vi "Intrinsic Imager.vi"() -> ()   [LabVIEW 2014]
uses:
  <vilib>/vision/Image Controls.llb/IMAQ Image.ctl
  <instrlib>/niHWS/nihws.llb/niHWS Open File Permissions ID.ctl
  <vilib>/Utility/error.llb/DialogType.ctl
  <vilib>/DAQmx/read.llb/DAQmx Read (Analog Wfm 1Chan NSamp).vi
  <vilib>/Analysis/baseanly.llb/Mean (DBL).vi
  <instrlib>/niHWS/nihws.llb/niHWS Write Analog DBL.vi
  <vilib>/DAQmx/miscellaneous.llb/DAQmx Fill In Error Info.vi
  <instrlib>/niHWS/nihws.llb/niHWS Write Analog WDT.vi
  <instrlib>/niHWS/nihws.llb/niHWS Write Digital 2D U16.vi
  <vilib>/vision/NI_Vision_Development_Module.lvlib
  <resource>/objmgr/daqmx.rc
  <vilib>/Analysis/NI_AALBase.lvlib
panel:
  in  "Single trial":bool
  in  "Analysis":enum32{"Amp", "Angle", "Amp/Angle"}(radio)
  in  "Analyze":bool
  in  "Period (ms)":dbl=16641.0
  in  "Pixel Thr":dbl=4095.0
  in  "Magnify":bool
  in  "PseudoColor":bool
  out "Frames":u32 caption="Image Number"
  out "Rep. Fps":dbl caption="Frame Rate"
  out "Fps":dbl
  out "Ephys Rate":dbl=1000.0
  in  "Final res.":dbl=512.0
  out "Image Parameters : Bits per Pixel":u32
  out "Numeric":i32
  out "Setup":i32
  out "PPhocus?":bool
  out "file handle out":u32
  out "Recording":bool
  in  "stop":bool
  out "Raw Image":T1(plugin-control)
  out "Rec Time":dbl
  out "Photodiode display":waveform(dbl)(graph)
  in  "Recording Path":path
  in  "Rec":bool
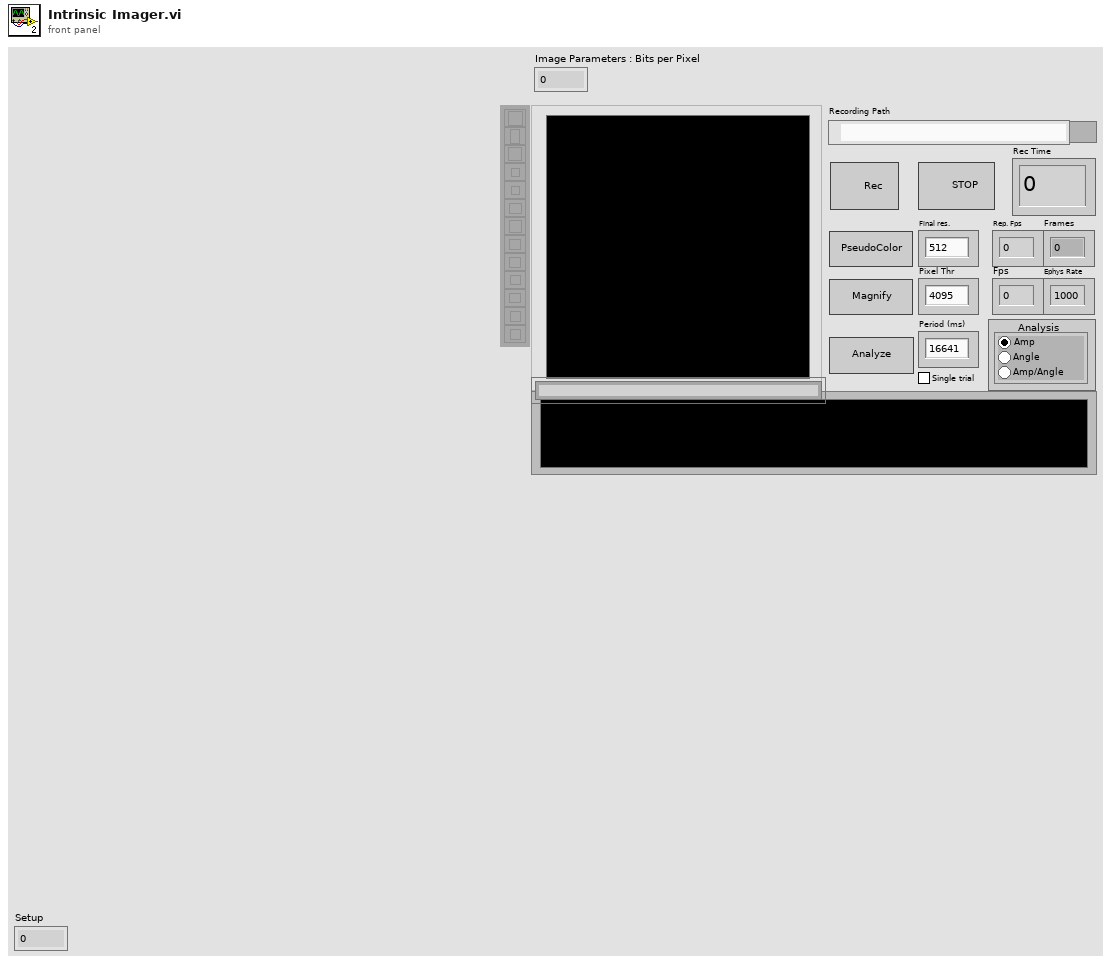
[diagram p1: front panel]
types:
  T1 = typedef "IMAQ Image.ctl" = refnum<image>
  T2 = typedef "niHWS Open File Permissions ID.ctl" = enum32{"Read Only", "Read/Write Existing", "Read/Write/Create New", "Read/Write/Create New Always"}
  T3 = enum32{"Average", "Min", "Max", "Clear  if < ", "Clear  if < or =", "Clear  if =", "Clear  if > or =", "Clear  if >"}
  T4 = enum32{"Invalid", "Standard", "Closed", "Hidden", "Minimized", "Maximized"}
  T5 = typedef "Image Type" = u32
  T6 = cluster{"IMAQ Session Out":refnum<k11>, "New Image":T1, "error out":errorcluster, cluster{dbl, i32}[], "New Image":T1}
  T7 = cluster{"IMAQ Session Out":refnum<k11>, "Image Out":T1, "error out":errorcluster, cluster{dbl, i32}[], "New Image":T1}
  T8 = typedef "DialogType.ctl" = u16
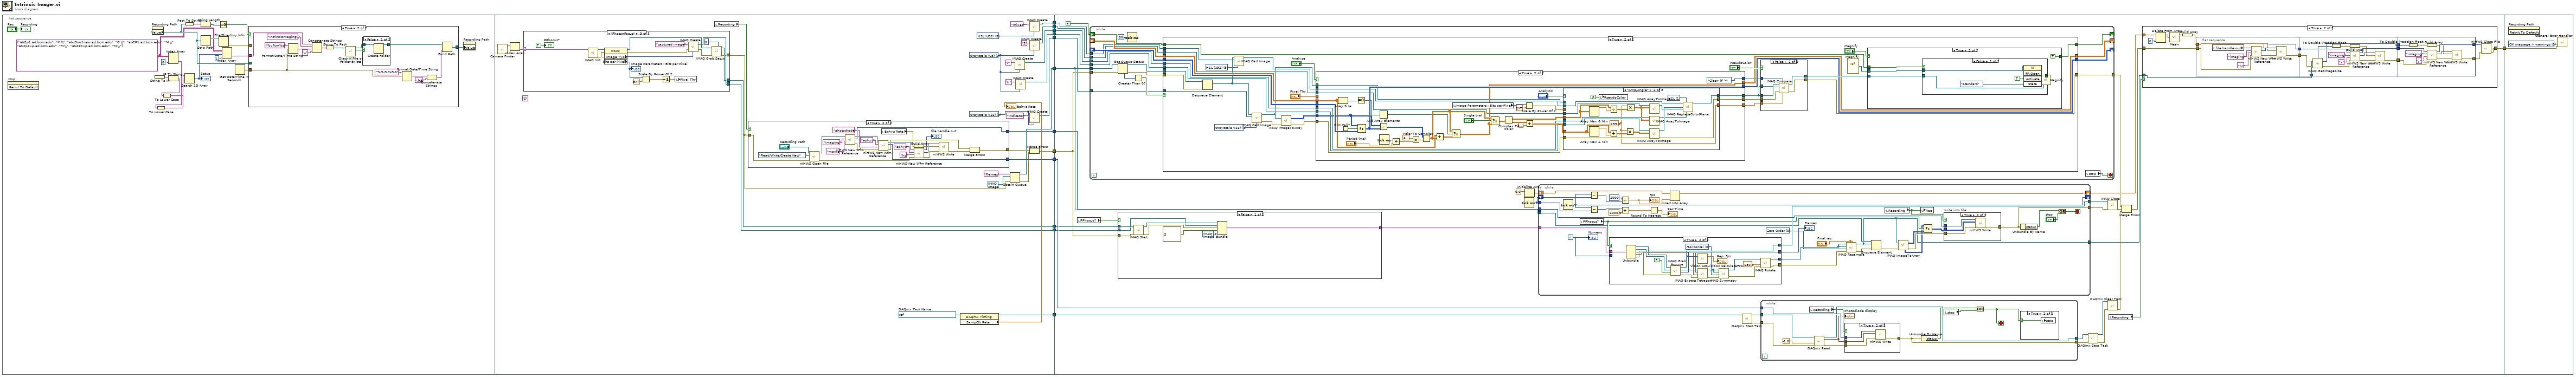
[diagram p0: block diagram]
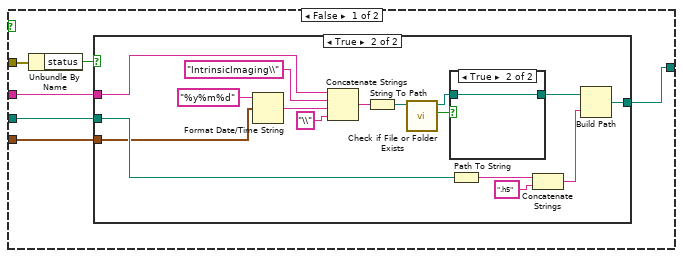
[diagram p2: hidden frame]
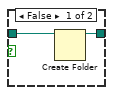
[diagram p4: hidden frame]
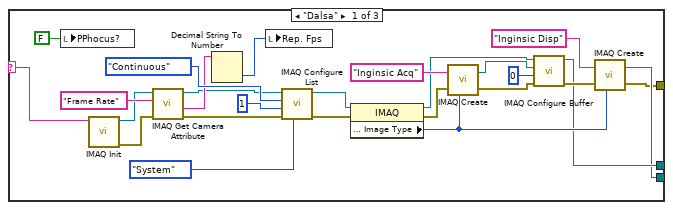
[diagram p6: hidden frame]
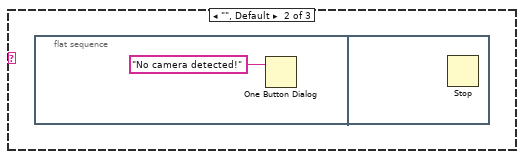
[diagram p7: hidden frame]
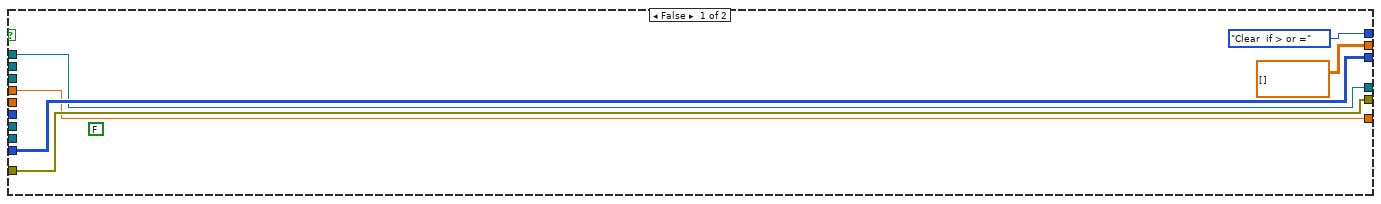
[diagram p10: hidden frame]
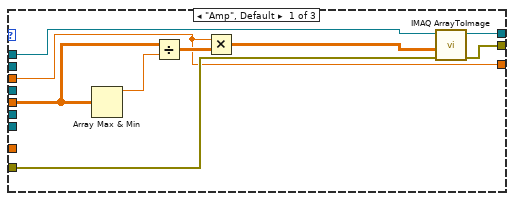
[diagram p11: hidden frame]
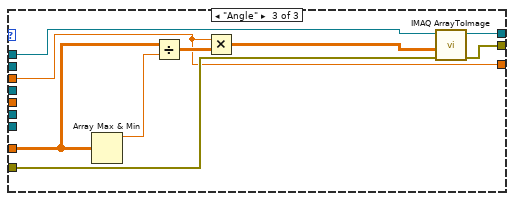
[diagram p12: hidden frame]
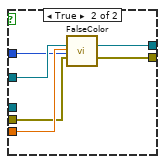
[diagram p13: hidden frame]
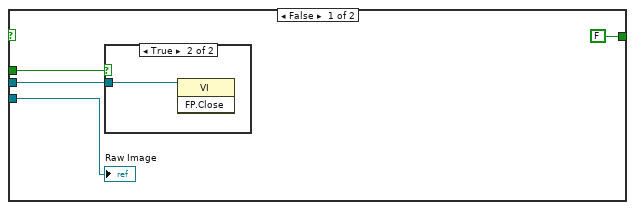
[diagram p14: hidden frame]
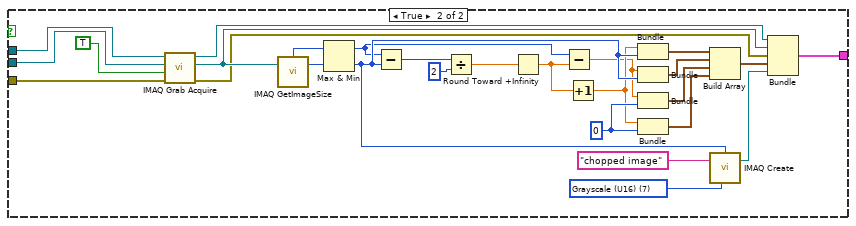
[diagram p17: hidden frame]
diagram:
  n1 = flat-sequence {
    tunnel: [w107] -> w13
    tunnel: [w106] -> w12
    tunnel: [w100] -> w10
    tunnel: [w104] -> w9
    tunnel: [w101] -> w8
    tunnel: [w92] -> w7
    tunnel: [w91] -> w6
    tunnel: [w88] -> w5
    tunnel: [w86] -> w4
    tunnel: [w84] -> w3
    tunnel: [w83] -> w2
    tunnel: [w79] -> w1
    tunnel: w13 -> [w203]
    tunnel: w12 -> [w204]
    tunnel: [w202] -> w11
    tunnel: w10 -> [w193]
    tunnel: w9 -> [w194]
    tunnel: w8 -> [w185]
    tunnel: w7 -> [w182]
    tunnel: w6 -> [w183]
    tunnel: w5 -> [w180]
    tunnel: w4 -> [w179]
    tunnel: w3 -> [w178]
    tunnel: w2 -> [w177]
    tunnel: w1 -> [w176]
    tunnel: w11 -> [w551]
    frame #0 {
      w19 = string[][] [["at-2p1.ad.bcm.edu", "M:\\"], ["at-s5no1new.ad.bcm.edu", "G:\\"], ["at-2P1.ad.bcm.edu", "M:\\"], ["at-2p1xp.ad.bcm.edu", "M:\\"], ["at-2P1xp.ad.bcm.edu", "M:\\"]]
      n2 = invoke on="stop" class="Bool (strict)" method="Reinit To Default"() -> ()  [unwired: 3 in, 3 out]
      n3 = property on="Recording Path" class="Path"() -> ("Value"=w26:path)  [unwired: 2 in, 2 out]
      n4 = String To IP() -> (0:w23:u32)  [unwired: 1 in]
      n5 = IP To String(2:w23) -> (0:w15:string)  [unwired: 1 in]
      n6 = To Lower Case(string=w15) -> (all lower case string=w14:string)
      n7 = Index Array(array=w19, index (col)=0 ("disabled index (col)")) -> (element=w17:string[])  [unwired: 1 in]
      n8 = To Lower Case(string=w17) -> (all lower case string=w16:string[])
      n9 = Path To String(path=w26) -> (string=w31:string)
      n10 = Search 1D Array(1D array=w16, element=w14) -> (index of element=w20:i32)  [unwired: 1 in]
      "Setup" <- w20
      n11 = String Length(string=w31) -> (length=w30:i32)
      n12 = Strip Path(path=w26) -> (stripped path=w25:path)  [unwired: 1 out]
      n13 = Equal To 0?(x=w30) -> (x = 0?=w29:bool)
      n14 = File/Directory Info(path=w25) -> (error out=w24:errorcluster)  [unwired: 1 in, 6 out]
      n15 = Index Array(array=w19, index (row)=w20, index (col)=1 ("disabled index (col)")) -> (element=w18:string)
      n16 = Get Date/Time In Seconds() -> (seconds since 1Jan1904=w32:timestamp)
      n17 = case shown="True" w29 {
        tunnel: w32 -> [w36 w65]
        tunnel: w26 -> [w37 _]
        tunnel: [w38 w63] -> w28
        tunnel: w24 -> [w34 _]
        tunnel: w18 -> [w33 w59]
        frame False {
          n18 = Unbundle By Name(w34) -> ("status"=w35:bool)
          n19 = case shown="True" w35 {
            tunnel: [w39 w46] -> w38
            tunnel: w37 -> [w39 w45]
            tunnel: w36 -> [_ w41]
            tunnel: w33 -> [_ w40]
            frame False {
            }
            frame True {
              n20 = Format Date/Time String(time format string (%c)="%y%m%d", seconds (now)=w41) -> (date/time string=w50:string)  [unwired: 1 in]
              n21 = Concatenate Strings(w40, "IntrinsicImaging\\", w50, "\\") -> (w49:string)
              n22 = String To Path(string=w49) -> (path=w55:path)
              n23 = call <vilib>:"Check if File or Folder Exists.vi"("path"=w55) -> ("file or folder exists?"=w53:bool, "dup path"=w52:path)  [unwired: 8 in, 1 out]
              n24 = case shown="True" w53 {
                tunnel: [w57 w58] -> w54
                tunnel: w52 -> [w56 w58]
                frame False {
                  n25 = Create Folder(path (use dialog)=w56) -> (created path=w57:path)  [unwired: 2 in, 2 out]
                }
                frame True {
                }
              }
              n26 = Path To String(path=w45) -> (string=w42:string)
              n27 = Concatenate Strings(w42, ".h5" ("string")) -> (w43:string)
              n28 = Build Path(base path=w54, name or relative path=w43) -> (appended path=w46:path)
            }
          }
        }
        frame True {
          n29 = Format Date/Time String(time format string (%c)="%y%m%d", seconds (now)=w65) -> (date/time string=w71:string)  [unwired: 1 in]
          n30 = Concatenate Strings(w59, "IntrinsicImaging\\", w71, "\\") -> (w72:string)
          n31 = String To Path(string=w72) -> (path=w64:path)
          n32 = call <vilib>:"Check if File or Folder Exists.vi"("path"=w64) -> ("file or folder exists?"=w68:bool, "dup path"=w69:path)  [unwired: 8 in, 1 out]
          n33 = case shown="False" w68 {
            tunnel: [w76 w77] -> w67
            tunnel: w69 -> [w75 w77]
            frame False {
              n34 = Create Folder(path (use dialog)=w75) -> (created path=w76:path)  [unwired: 2 in, 2 out]
            }
            frame True {
            }
          }
          n35 = Format Date/Time String(time format string (%c)="%H-%M-%S", seconds (now)=w65) -> (date/time string=w62:string)  [unwired: 1 in]
          n36 = Concatenate Strings(w62, ".h5" ("string")) -> (w60:string)
          n37 = Build Path(base path=w67, name or relative path=w60) -> (appended path=w63:path)
        }
      }
      n38 = property on="Recording Path" class="Path"("Value"=w28) -> ()  [unwired: 2 in, 2 out]
      "Recording" <- "Rec"
    }
    frame #1 {
      w80 = T5 1 items=["Grayscale (U8)", "Grayscale (I16)", "Grayscale (SGL)", "Complex (CSG)", "RGB (U32)", "HSL (U32)", "RGB (U64)", "Grayscale (U16)"] ("Image Type")
      (unwired) "S" ("Image Name")
      w82 = T5 0 items=["Grayscale (U8)", "Grayscale (I16)", "Grayscale (SGL)", "Complex (CSG)", "RGB (U32)", "HSL (U32)", "RGB (U64)", "Grayscale (U16)"] ("Image Type")
      w89 = T5 5 items=["Grayscale (U8)", "Grayscale (I16)", "Grayscale (SGL)", "Complex (CSG)", "RGB (U32)", "HSL (U32)", "RGB (U64)", "Grayscale (U16)"] ("Image Type")
      w103 = refnum<k21> "Photodiode Intrinsic Imaging"  # DAQmx Task Name
      n39 = call "Camera Finder.vi"() -> ("IMAQ Interfaces"=w98:string[])  [unwired: 11 in]
      n40 = Index Array(array=w98) -> (element=w99:string)  [unwired: 1 in]
      n41 = case shown="\"PhotonFocus\"" w99 {
        selector: w99 -> [w111 _ w140]
        tunnel: [w114 _ w143] -> w104
        tunnel: [w115 _ w142] -> w100
        tunnel: [w113 _ w141] -> w95
        frame "Dalsa" {
          n42 = local write "PPhocus?"(FALSE ("PPhocus?")) -> ()
          n43 = call <vilib>:"IMAQ Init.vi"("Interface Name"=w111) -> ("error out"=w116:errorcluster, "IMAQ Session Out"=w117:refnum<k11>)  [unwired: 9 in]
          n44 = call <vilib>:"IMAQ Get Camera Attribute.vi"("error in (no error)"=w116, "Camera Attribute"="Frame Rate", "IMAQ Session In"=w117) -> ("error out"=w108:errorcluster, "Attribute Value"=w110:string, "IMAQ Session Out"=w109:refnum<k11>)  [unwired: 4 in]
          n45 = Decimal String To Number(string=w110) -> (number=w112:i32)  [unwired: 2 in, 1 out]
          n46 = local write "Rep. Fps"(w112) -> ()
          n47 = call <vilib>:"IMAQ Configure List.vi"("Memory Location"=enum16{"System", "Onboard"}."System", "error in (no error)"=w108, "Number of buffers"=u32 1, "Continuous?"=enum16{"One-Shot", "Continuous"}."Continuous" ("Continuous ?"), "IMAQ Session In"=w109) -> ("error out"=w125:errorcluster, "IMAQ Session Out"=w126:refnum<k11>)  [unwired: 5 in]
          n48 = property class="IMAQ"(reference=w126, error in=w125) -> (reference out=w124:refnum<k11>, error out=w123:errorcluster, "Image Parameters : Image Type"=w122:u32)
          n49 = call "IMAQ Create"("Image Name"="Inginsic Acq", "Image Type"=w122, "error in (no error)"=w123) -> ("New Image"=w119:T1, "error out"=w129:errorcluster)  [unwired: 2 in]
          n50 = call <vilib>:"IMAQ Configure Buffer.vi"("error in (no error)"=w129, "Buffer Number"=u32 0, "Image In"=w119, "IMAQ Session In"=w124) -> ("error out"=w121:errorcluster, "IMAQ Session Out"=w115:refnum<k11>)  [unwired: 6 in]
          n51 = call "IMAQ Create"("Image Name"="Inginsic Disp", "Image Type"=w122, "error in (no error)"=w121) -> ("New Image"=w114:T1, "error out"=w113:errorcluster)  [unwired: 2 in]
        }
        frame "", Default {
          n52 = flat-sequence {
            frame #0 {
              n53 = One Button Dialog(message="No camera detected!" ("error source (\" \")")) -> ()  [unwired: 1 in, 1 out]
            }
            frame #1 {
              n54 = Stop() -> ()  [unwired: 1 in]
            }
          }
        }
        frame "PhotonFocus" {
          n55 = call <vilib>:"IMAQ Init.vi"("Interface Name"=w140) -> ("error out"=w150:errorcluster, "IMAQ Session Out"=w149:refnum<k11>)  [unwired: 1 in, 8 out]
          n56 = property class="IMAQ"(reference=w149, error in=w150) -> (reference out=w144:refnum<k11>, error out=w147:errorcluster, "Image Parameters : Image Type"=w148:u32, "Bits per Pixel"=w138:u32)
          "Image Parameters : Bits per Pixel" <- w138
          n57 = Scale By Power Of 2(n=w138, x=ext 1.0) -> (x*2^n=w136:ext)
          n58 = Decrement(x=w136) -> (x-1=w135:ext)
          n59 = local write "Pixel Thr"(w135) -> ()
          n60 = call "IMAQ Create"("Image Name"="captured image", "Image Type"=w148, "error in (no error)"=w147) -> ("New Image"=w143:T1, "error out"=w145:errorcluster)  [unwired: 1 in, 1 out]
          n61 = call <vilib>:"IMAQ Grab Setup.vi"("Channel"=0, "error in (no error)"=w145, "IMAQ Session In"=w144) -> ("error out"=w141:errorcluster, "IMAQ Session Out"=w142:refnum<k11>)  [unwired: 7 out]
          "PPhocus?" <- TRUE ("PPhocus?")
        }
      }
      n62 = local read "Recording"() -> (w105:bool)
      n63 = case shown="True" w105 {
        tunnel: [_ w175] -> w107
        tunnel: [_ w155] -> w94
        tunnel: [_ w173] -> w106
        tunnel: w95 -> [_ w152]
        frame False {
        }
        frame True {
          n64 = call <instrlib>:"niHWS Open File.vi"("error in (no error)"=w152, "permissions (0:read only)"=niHWS_Open_File_Permissions_ID."Read/Write/Create New", "file path"="Recording Path") -> ("error out"=w170:errorcluster, "file handle"=w162:u32)  [unwired: 7 in]
          n65 = call <instrlib>:"niHWS New Wfm Reference.vi"("waveform name (empty)"="movie" ("format string"), "group name (empty)"="imaging", "file handle in"=w162) -> ("error out"=w158:errorcluster, "waveform reference"=w175:u32, "file handle out"=w159:u32)  [unwired: 6 in]
          n66 = call <instrlib>:"niHWS New Wfm Reference.vi"("error in (no error)"=w158, "waveform name (empty)"="photodiode", "group name (empty)"="ephys", "file handle in"=w159) -> ("error out"=w157:errorcluster, "waveform reference"=w173:u32, "file handle out"=w174:u32)  [unwired: 5 in]
          n67 = local read "Ephys Rate"() -> (w153:dbl)
          n68 = Build Array(w153) -> (w166:dbl[])
          n69 = call <instrlib>:"niHWS New Wfm Reference.vi"("error in (no error)"=w170, "waveform name (empty)"="hz" ("group name (empty)"), "group name (empty)"="ephys", "file handle in"=w174) -> ("error out"=w165:errorcluster, "waveform reference"=w169:u32, "file handle out"=→"file handle out":u32)  [unwired: 5 in]
          n70 = call-poly <instrlib>:"niHWS Write.vi"("error in (no error)"=w165, "data"=w166, "waveform reference in"=w169) -> ("error out"=w156:errorcluster)  [unwired: 7 in, 1 out]
          n71 = Merge Errors(w157, w156) -> (w155:errorcluster)
        }
      }
      n72 = property class="DAQmx Timing"(reference=w103) -> (reference out=w101:refnum<k21>, "SampClk.Rate"=→"Ephys Rate":dbl)  [unwired: 1 in, 1 out]
      n73 = Obtain Queue(name (unnamed)="Frames", element data type=T1 refnum ("New Image"), error in (no error)=w95) -> (queue out=w91:refnum<queue>, error out=w93:errorcluster)  [unwired: 2 in, 1 out]
      n74 = call "IMAQ Create"("Image Name"="V", "Image Type"=w82) -> ("New Image"=w86:T1)  [unwired: 3 in, 1 out]
      n75 = call "IMAQ Create"("Image Name"="H", "Image Type"=w82) -> ("New Image"=w84:T1)  [unwired: 3 in, 1 out]
      n76 = call "IMAQ Create"("Image Name"="mixed", "Image Type"=w89) -> ("New Image"=w88:T1)  [unwired: 3 in, 1 out]
      n77 = call "IMAQ Create"("Image Name"="S", "Image Type"=w82) -> ("New Image"=w83:T1)  [unwired: 3 in, 1 out]
      n78 = call "IMAQ Create"("Image Name"="Indicator", "Image Type"=w80) -> ("New Image"=w79:T1)  [unwired: 3 in, 1 out]
      n79 = Merge Errors(w94, w93) -> (w92:errorcluster)
    }
    frame #2 {
      n80 = local read "PPhocus?"() -> (w187:bool)
      n81 = while {
        shift-right: [w228] -> _
        shift-left: FALSE -> [w227]
        tunnel: w183 -> [w225]
        tunnel: w182 -> [w221]
        tunnel: [w219] -> w181
        shift-right: [w218] -> _
        shift-left: _ -> [w217]
        shift-right: [w216] -> _
        shift-left: _ -> [w215]
        tunnel: w180 -> [w214]
        tunnel: w179 -> [w213]
        tunnel: w178 -> [w212]
        tunnel: w177 -> [w211]
        tunnel: w176 -> [w210]
        stop <- w229 stop-if-true
        n82 = Get Queue Status(queue=w225, error in (no error)=w221) -> (queue out=w222:refnum<queue>, error out=w220:errorcluster, # elements in queue=w224:i32)  [unwired: 1 in, 5 out]
        n83 = Wait (ms)(milliseconds to wait=u32 50) -> ()  [unwired: 1 out]
        n84 = Greater Than 0?(x=w224) -> (x > 0?=w223:bool)
        n85 = case shown="True" w223 {
          tunnel: [w233 w263] -> w228
          tunnel: w227 -> [w233 w262]
          tunnel: w222 -> [_ w259]
          tunnel: w220 -> [w232 w258]
          tunnel: [w232 w256] -> w219
          tunnel: [w231 w254] -> w218
          tunnel: w217 -> [w231 w253]
          tunnel: [w230 w252] -> w216
          tunnel: w215 -> [w230 w251]
          tunnel: w214 -> [_ w238]
          tunnel: w213 -> [_ w237]
          tunnel: w212 -> [_ w236]
          tunnel: w211 -> [_ w235]
          tunnel: w210 -> [_ w234]
          frame False {
          }
          frame True {
            w240 = T5 5 items=["Grayscale (U8)", "Grayscale (I16)", "Grayscale (SGL)", "Complex (CSG)", "RGB (U32)", "HSL (U32)", "RGB (U64)", "Grayscale (U16)"] ("Image Type")
            w242 = T5 1 items=["Grayscale (U8)", "Grayscale (I16)", "Grayscale (SGL)", "Complex (CSG)", "RGB (U32)", "HSL (U32)", "RGB (U64)", "Grayscale (U16)"] ("Image Type")
            n86 = Dequeue Element(queue=w259, error in (no error)=w258) -> (element=w241:T1)  [unwired: 1 in, 3 out]
            n87 = call "IMAQ Cast Image"("Image Type"=w240, "Image Dst"=w238, "Image Src"=w241) -> ("Image Dst Out"=w239:T1)  [unwired: 7 in, 1 out]
            n88 = call "IMAQ Cast Image"("Image Type"=w242, "Image Dst"=w234, "Image Src"=w241) -> ("error out"=w248:errorcluster, "Image Dst Out"=w250:T1)  [unwired: 7 in]
            n89 = call "IMAQ ImageToArray"("error in (no error)"=w248, "Image"=w250) -> ("error out"=w247:errorcluster, "Image Pixels (I16)"=w255:i16[][])  [unwired: 2 in, 3 out]
            n90 = case shown="True" "Analyze" {
              tunnel: w255 -> [w271 w306]
              tunnel: [w271 w305] -> w254
              tunnel: w253 -> [_ w307]
              tunnel: [cdb[][] [] w276] -> w252
              tunnel: w251 -> [_ w280]
              tunnel: w250 -> [w270 w295]
              tunnel: [w270 w294] -> w249
              tunnel: w247 -> [w269 w292]
              tunnel: [w269 w293] -> w246
              tunnel: [w268 w286] -> w245
              tunnel: "Pixel Thr" -> [w268 _]
              tunnel: [T3."Clear  if > or =" ("Operator") T3."Clear  if >" ("Operator")] -> w243
              tunnel: w239 -> [_ w275]
              tunnel: w236 -> [_ w274]
              tunnel: w235 -> [_ w273]
              tunnel: w237 -> [_ w272]
              frame False {
                (unwired) FALSE
              }
              frame True {
                n91 = Array Size(array=w280) -> (size(s)=w279:i32[])
                n92 = First Call?() -> (First Call?: T/F=w308:bool)
                n93 = Equal To 0?(x=w279) -> (x = 0?=w278:bool[])
                n94 = Select(t=w306, s=w308, f=w307) -> (s? t:f=w305:i16[][])
                n95 = And Array Elements(Boolean array=w278) -> (logical AND=w277:bool)
                n96 = Subtract(x=w306, y=w305) -> (x-y=w299:i16[][])
                n97 = Tick Count (ms)() -> (millisecond timer value=w302:u32)
                n98 = Divide(x=w302, y="Period (ms)") -> (x/y=w300:dbl)
                n99 = Multiply(x=6.283185307179586, y=w300) -> (x*y=w304:dbl)
                n100 = Polar To Complex(1:w304, 2:w299) -> (0:w281:cdb[][])
                n101 = Add(x=w280, y=w281) -> (x+y=w282:cdb[][])
                n102 = Select(t=w281, s=w277, f=w282) -> (s? t:f=w276:cdb[][])
                n103 = local read "Image Parameters : Bits per Pixel"() -> (w288:u32)
                n104 = Select(t=w281, s="Single trial", f=w276) -> (s? t:f=w283:cdb[][])
                n105 = Complex To Polar(r * e^(i*theta)=w283) -> (r=w291:dbl[][], theta=w298:dbl[][])
                n106 = Scale By Power Of 2(n=w288, x=ext 1.0) -> (x*2^n=w287:ext)
                n107 = Add(x=w298, y=3.141592653589793) -> (x+y=w290:dbl[][])
                n108 = case shown="\"Amp/Angle\"" "Analysis" {
                  tunnel: w295 -> [w309 _ w344]
                  tunnel: [w315 w330 w341] -> w294
                  tunnel: [w314 w333 w342] -> w293
                  tunnel: w292 -> [w313 w334 w343]
                  tunnel: w291 -> [w312 w318 _]
                  tunnel: w290 -> [_ w319 w345]
                  tunnel: w287 -> [w311 _ w340]
                  tunnel: [w311 w320 w340] -> w286
                  tunnel: w275 -> [_ w331 _]
                  tunnel: w274 -> [_ w326 _]
                  tunnel: w273 -> [_ w325 _]
                  tunnel: w272 -> [_ w323 _]
                  frame "Amp", Default {
                    n109 = Array Max & Min(array=w312) -> (max value=w316:dbl)  [unwired: 3 out]
                    n110 = Divide(x=w312, y=w316) -> (x/y=w317:dbl[][])
                    n111 = Multiply(x=w311, y=w317) -> (x*y=w310:ext[][])
                    n112 = call "IMAQ ArrayToImage"("error in (no error)"=w313, "Image Pixels (I16)"=w310, "Image"=w309) -> ("error out"=w314:errorcluster, "Image Out"=w315:T1)  [unwired: 7 in]
                  }
                  frame "Amp/Angle" {
                    w332 = u16 1 items=["RGB", "HSL", "HSV", "HSI"] ("Color Mode")
                    w320 = 255.0
                    n113 = Array Max & Min(array=w318) -> (max value=w336:dbl)  [unwired: 3 out]
                    n114 = Array Max & Min(array=w319) -> (max value=w337:dbl)  [unwired: 3 out]
                    n115 = local write "PseudoColor"(FALSE ("PseudoColor")) -> ()
                    n116 = Divide(x=w318, y=w336) -> (x/y=w335:dbl[][])
                    n117 = Divide(x=w319, y=w337) -> (x/y=w338:dbl[][])
                    n118 = Multiply(x=w320, y=w338) -> (x*y=w328:dbl[][])
                    n119 = Multiply(x=w320, y=w335) -> (x*y=w322:dbl[][])
                    n120 = call "IMAQ ArrayToImage"("Image Pixels (U8)"=w322, "Image"=w325) -> ("Image Out"=w324:T1)  [unwired: 8 in, 1 out]
                    n121 = call "IMAQ ArrayToImage"("Image Pixels (U8)"=w322, "Image"=w323) -> ("Image Out"=w321:T1)  [unwired: 8 in, 1 out]
                    n122 = call "IMAQ ArrayToImage"("error in (no error)"=w334, "Image Pixels (U8)"=w328, "Image"=w326) -> ("error out"=w333:errorcluster, "Image Out"=w327:T1)  [unwired: 7 in]
                    n123 = call "IMAQ ReplaceColorPlane"("Image Src"=w331, "Color Mode"=w332, "Red or Hue Plane"=w327, "Green or Sat Plane"=w324, "Blue or Luma or Val or Inten Plane"=w321) -> ("Image Dst Out"=w330:T1)  [unwired: 9 in, 1 out]
                  }
                  frame "Angle" {
                    n124 = Array Max & Min(array=w345) -> (max value=w346:dbl)  [unwired: 3 out]
                    n125 = Divide(x=w345, y=w346) -> (x/y=w347:dbl[][])
                    n126 = Multiply(x=w340, y=w347) -> (x*y=w339:ext[][])
                    n127 = call "IMAQ ArrayToImage"("error in (no error)"=w343, "Image Pixels (I16)"=w339, "Image"=w344) -> ("error out"=w342:errorcluster, "Image Out"=w341:T1)  [unwired: 7 in]
                  }
                }
              }
            }
            n128 = case shown="False" "PseudoColor" {
              tunnel: w249 -> [w354 w360]
              tunnel: w249 -> [w353 _]
              tunnel: w243 -> [w352 w355]
              tunnel: w245 -> [w351 w358]
              tunnel: [w350 w359] -> w261
              tunnel: w246 -> [w349 w357]
              tunnel: [w348 w356] -> w256
              frame False {
                n129 = call "IMAQ Compare"("Constant"=w351, "Operator"=w352, "error in (no error)"=w349, "Image Dst"=w353, "Image Src A"=w354) -> ("error out"=w348:errorcluster, "Image Dst Out"=w350:T1)  [unwired: 5 in]
              }
              frame True {
                n130 = call "FalseColor.vi"("Image"=w360, "maxValue"=w358, "Operator"=w355, "error in (no error)"=w357) -> ("Image Dst Out"=w359:T1, "error out"=w356:errorcluster)  [unwired: 22 in]
              }
            }
            n131 = vi-ref "Magnify.vi"() -> (w265:refnum<vi>)
            n132 = case shown="True" "Magnify" {
              tunnel: w265 -> [w364 w370]
              tunnel: [FALSE TRUE] -> w263
              tunnel: w262 -> [w363 w368]
              tunnel: w261 -> [w361 w367]
              frame False {
                n133 = case shown="True" w363 {
                  tunnel: w364 -> [_ w365]
                  frame False {
                  }
                  frame True {
                    n134 = invoke class="VI" method="FP.Close"(reference=w365) -> ()  [unwired: 2 in, 3 out]
                  }
                }
                "Raw Image" <- w361
              }
              frame True {
                n135 = case shown="False" w368 {
                  tunnel: w370 -> [w373 _]
                  tunnel: w367 -> [w371 w375]
                  tunnel: [w371 w375] -> w366
                  frame False {
                    n136 = invoke class="VI" method="FP.Open"(reference=w373, "Activate"=TRUE ("Wait Until Done"), "State"=T4."Standard") -> ()  [unwired: 2 in, 5 out]
                  }
                  frame True {
                  }
                }
                n137 = call "Magnify.vi"("Camera 2"=w366) -> ()  [unwired: 11 in]
              }
            }
          }
        }
        n138 = local read "stop"() -> (w229:bool)
      }
      n139 = case shown="False" w187 {
        tunnel: w194 -> [w379 w408]
        tunnel: w182 -> [w381 w407]
        tunnel: w193 -> [w382 w406]
        tunnel: [w383 w386] -> w186
        frame False {
          n140 = call <vilib>:"IMAQ Start.vi"("error in (no error)"=w381, "IMAQ Session In"=w382) -> ("error out"=w378:errorcluster, "IMAQ Session Out"=w380:refnum<k11>)  [unwired: 8 in]
          n141 = Bundle("IMAQ Session Out"=w380, "New Image"=w379, "error out"=w378, cluster{dbl, i32}[] [], "New Image"=T1 refnum) -> (w383:T6)  [unwired: 1 in]
        }
        frame True {
          w402 = 0
          w409 = T5 7 items=["Grayscale (U8)", "Grayscale (I16)", "Grayscale (SGL)", "Complex (CSG)", "RGB (U32)", "HSL (U32)", "RGB (U64)", "Grayscale (U16)"] ("Image Type")
          n142 = call <vilib>:"IMAQ Grab Acquire.vi"("error in (no error)"=w407, "Immediate?"=TRUE, "Image In"=w408, "IMAQ Session In"=w406) -> ("error out"=w387:errorcluster, "Image Out"=w388:T1, "IMAQ Session Out"=w389:refnum<k11>)  [unwired: 5 out]
          n143 = call "IMAQ GetImageSize"("Image"=w388) -> ("Y Resolution"=w403:i32, "X Resolution"=w404:i32)  [unwired: 3 in, 1 out]
          n144 = Max & Min(x=w404, y=w403) -> (max(x,y)=w395:i32, min(x,y)=w401:i32)
          n145 = Subtract(x=w395, y=w401) -> (x-y=w400:i32)
          n146 = Divide(x=w400, y=2) -> (x/y=w398:dbl)
          n147 = Round Toward +Infinity(x=w398) -> (ceil(x): smallest int >= x=w396:dbl)
          n148 = Subtract(x=w395, y=w396) -> (x-y=w394:dbl)
          n149 = Increment(x=w396) -> (x+1=w397:dbl)
          n150 = Bundle(w397, w401) -> (w390:cluster{dbl, i32})  [unwired: 1 in]
          n151 = Bundle(w394, w401) -> (w393:cluster{dbl, i32})  [unwired: 1 in]
          n152 = Bundle(w394, w402) -> (w392:cluster{dbl, i32})  [unwired: 1 in]
          n153 = Bundle(w397, w402) -> (w391:cluster{dbl, i32})  [unwired: 1 in]
          n154 = Build Array(w390, w393, w392, w391) -> (w385:cluster{dbl, i32}[])
          n155 = call "IMAQ Create"("Border Size"=w401, "Image Name"="chopped image", "Image Type"=w409) -> ("New Image"=w384:T1)  [unwired: 1 in, 2 out]
          n156 = Bundle("IMAQ Session Out"=w389, "Image Out"=w388, "error out"=w387, w385, "New Image"=w384) -> (w386:T7)  [unwired: 1 in]
        }
      }
      n157 = Tick Count (ms)() -> (millisecond timer value=w209:u32)
      n158 = Initialize Array(0.0 ("element")) -> (w200:dbl[])  [unwired: 1 in]
      n159 = while {
        tunnel: w203 -> [w513]
        shift-right: [w508] -> _
        shift-left: w209 -> [w512]
        tunnel: w209 -> [w507]
        shift-right: [w501] -> w198
        shift-left: w200 -> [w502]
        tunnel: [w497] -> w190
        tunnel: [w487] -> w197
        tunnel: [w479] -> w192
        tunnel: w186 -> [w489]
        tunnel: w183 -> [w482]
        i -> [w490]
        stop <- w498 stop-if-true
        w488 = u32 0 items=["Zero Order", "Bi-Linear", "Quadratic", "Cubic Spline"] ("Interpolation Type")
        n160 = Tick Count (ms)() -> (millisecond timer value=w508:u32)
        n161 = local read "PPhocus?"() -> (w486:bool)
        n162 = Subtract(x=w508, y=w512) -> (x-y=w511:u32)
        n163 = Subtract(x=w508, y=w507) -> (x-y=w506:u32)
        n164 = case shown="True" w486 {
          tunnel: [w520 w544] -> w487
          tunnel: [w519 w528] -> w493
          tunnel: [w518 w527] -> w492
          tunnel: [w525 w539] -> w491
          tunnel: w490 -> [w525 _]
          tunnel: w489 -> [w524 w538]
          frame False {
            n165 = local read "Rep. Fps"() -> (w517:dbl)
            n166 = Reciprocal(x=w517) -> (1/x=w516:dbl)
            n167 = Multiply(x=1000.0, y=w516) -> (x*y=w514:dbl)
            n168 = Wait (ms)(milliseconds to wait=w514) -> ()  [unwired: 1 out]
            n169 = Unbundle(w524) -> ("IMAQ Session Out"=w523:refnum<k11>, "Image Out"=w522:T1, "error out"=w521:errorcluster)  [unwired: 2 out]
            n170 = call <vilib>:"IMAQ Copy Acquired Buffer.vi"("IMAQ Session In"=w523, "Image In"=w522, "error in (no error)"=w521) -> ("IMAQ Session Out"=w520:refnum<k11>, "Image Out"=w519:T1, "error out"=w518:errorcluster)  [unwired: 8 in, 2 out]
          }
          frame True {
            w543 = u32 0 items=["Horizontal", "Vertical", "Central", "1st Diagonal", "2nd Diagonal"] ("Type of Symmetry")
            n171 = Unbundle(w538) -> ("IMAQ Session Out"=w537:refnum<k11>, "Image Out"=w536:T1, "error out"=w535:errorcluster, w534:cluster{dbl, i32}[], "New Image"=w533:T1)
            n172 = call <vilib>:"IMAQ Grab Acquire.vi"("error in (no error)"=w535, "Immediate?"=FALSE, "Image In"=w536, "IMAQ Session In"=w537) -> ("error out"=w542:errorcluster, "Acquired Buffer Number"=w539:u32, "Image Out"=w532:T1, "IMAQ Session Out"=w544:refnum<k11>)  [unwired: 4 out]
            n173 = call <vilib>:"Vision Acquisition CalculateFPS.vi"("buffer number"=w539) -> ("acquired FPS"=→"Rep. Fps":dbl)  [unwired: 2 out]
            n174 = call-poly "IMAQ Extract Tetragon"("error in (no error)"=w542, "Tetragon"=w534, "Image Dst"=w533, "Image Src"=w532) -> ("error out"=w541:errorcluster, "Image Dst Out"=w540:T1)  [unwired: 6 in]
            n175 = call "IMAQ Symmetry"("error in (no error)"=w541, "Type of Symmetry"=w543, "Image Dst"=w540, "Image Src"=w540) -> ("error out"=w529:errorcluster, "Image Dst Out"=w530:T1)  [unwired: 1 in]
            n176 = call "IMAQ Rotate"("error in (no error)"=w529, "Angle (degrees)"=sgl 180.0, "Image Src"=w530) -> ("error out"=w527:errorcluster, "Image Dst Out"=w528:T1)  [unwired: 7 in]
          }
        }
        "Frames" <- w491
        n177 = Divide(x=u32 1000, y=w511) -> (x/y=w503:dbl)
        "Fps" <- w503
        n178 = Divide(x=w506, y=1000.0) -> (x/y=w505:dbl)
        n179 = Round To Nearest(number=w505) -> (nearest integer value=→"Rec Time":dbl)
        n180 = Insert Into Array(array=w502, new element=w503) -> (w501:dbl[])  [unwired: 1 in]
        n181 = call "IMAQ Resample"("X Resolution"="Final res.", "Y Resolution"="Final res.", "error in (no error)"=w492, "Interpolation Type"=w488, "Image Dst"=w493, "Image Src"=w493) -> ("error out"=w481:errorcluster, "Image Dst Out"=w479:T1)  [unwired: 4 in]
        n182 = Enqueue Element(queue=w482, element=w479, error in (no error)=w481) -> (error out=w480:errorcluster)  [unwired: 1 in, 2 out]
        n183 = local read "Recording"() -> (w494:bool)
        n184 = call "IMAQ ImageToArray"("error in (no error)"=w480, "Image"=w479) -> ("Image Pixels (U16)"=w483:u16[][], "error out"=w496:errorcluster, "Image Pixels (I16)"=w485:i16[][])  [unwired: 2 in, 2 out]
        n185 = local write "Rec"(w494) -> ()
        n186 = Select(t=w483, s=w486, f=w485) -> (s? t:f=w484:u16[][])
        n187 = case "write into file" shown="True" w494 {
          tunnel: w496 -> [w546 w549]
          tunnel: w484 -> [_ w550]
          tunnel: [w546 w548] -> w497
          tunnel: w513 -> [_ w547]
          frame False {
          }
          frame True {
            n188 = call-poly <instrlib>:"niHWS Write.vi"("error in (no error)"=w549, "data"=w550, "waveform reference in"=w547) -> ("error out"=w548:errorcluster)  [unwired: 7 in, 1 out]
          }
        }
        n189 = Unbundle By Name(w497) -> ("status"=w495:bool)
        n190 = Or(x=w495, y="stop") -> (x .or. y?=w498:bool)
        "Numeric" <- w490
      }
      n191 = call <vilib>:"DAQmx Start Task.vi"("task/channels in"=w185) -> ("task out"=w207:refnum<k21>, "error out"=w201:errorcluster)  [unwired: 13 in]
      n192 = while {
        tunnel: w207 -> [w472]
        tunnel: w201 -> [w468]
        tunnel: w204 -> [w471]
        tunnel: [w465] -> w191
        tunnel: [w469] -> w208
        stop <- w461 stop-if-true
        n193 = local read "Recording"() -> (w466:bool)
        n194 = call-poly <vilib>:"DAQmx Read.vi"("task/channels in"=w472, "timeout"=-1.0, "error in"=w468) -> ("task out"=w469:refnum<k21>, "data"=w470:waveform(dbl), "error out"=w464:errorcluster)  [unwired: 10 in]
        "Photodiode display" <- w470
        n195 = case shown="True" w466 {
          tunnel: w470 -> [_ w475]
          tunnel: w471 -> [_ w478]
          tunnel: [w474 w477] -> w465
          tunnel: w464 -> [w474 w476]
          frame False {
          }
          frame True {
            n196 = call-poly <instrlib>:"niHWS Write.vi"("error in (no error)"=w476, "analog waveform"=w475, "waveform reference in"=w478) -> ("error out"=w477:errorcluster)  [unwired: 7 in, 1 out]
          }
        }
        n197 = Unbundle By Name(w465) -> ("status"=w462:bool)
        n198 = local read "stop"() -> (w467:bool)
        n199 = Or(x=w462, y=w467) -> (x .or. y?=w461:bool)
        n200 = case shown="True" w461 {
          selector: w461 -> [_ w473]
          frame False {
          }
          frame True {
            n201 = local write "stop"(w473) -> ()
          }
        }
      }
      n202 = call <vilib>:"DAQmx Stop Task.vi"("task/channels in"=w208, "error in"=w191) -> ("task out"=w205:refnum<k21>, "error out"=w206:errorcluster)  [unwired: 12 in]
      n203 = call <vilib>:"IMAQ Close.vi"("error in (no error)"=w190, "IMAQ Session In"=w197) -> ("error out"=w196:errorcluster)  [unwired: 9 out]
      n204 = call <vilib>:"DAQmx Clear Task.vi"("task in"=w205, "error in"=w206) -> ("error out"=w189:errorcluster)  [unwired: 13 in]
      n205 = local read "Recording"() -> (w188:bool)
      n206 = Merge Errors(w181, w196, w189) -> (w195:errorcluster)
      n207 = case shown="True" w188 {
        tunnel: [w411 w426] -> w202
        tunnel: w198 -> [_ w425]
        tunnel: w195 -> [w411 w412]
        tunnel: w192 -> [_ w413]
        frame False {
        }
        frame True {
          n208 = Delete From Array(array=w425, index=0) -> (array with subset deleted=w423:dbl[])  [unwired: 1 in, 1 out]
          n209 = call-poly <vilib>:"Mean.vi"("X"=w423) -> ("mean"=w424:dbl)  [unwired: 1 out]
          n210 = Build Array(w424) -> (w419:dbl[])
          n211 = flat-sequence {
            tunnel: w419 -> [w430]
            tunnel: [w435] -> w421
            tunnel: [w429] -> w420
            tunnel: w412 -> [w428]
            tunnel: w421 -> [w437]
            tunnel: w420 -> [w446]
            tunnel: [w445] -> w418
            tunnel: [w443] -> w416
            tunnel: [w439] -> w414
            tunnel: w413 -> [w436]
            tunnel: w418 -> [w457]
            tunnel: [w456] -> w417
            tunnel: w416 -> [w455]
            tunnel: [w453] -> w415
            tunnel: w414 -> [w450]
            frame #0 {
              n212 = local read "file handle out"() -> (w427:u32)
              n213 = call <instrlib>:"niHWS New Wfm Reference.vi"("error in (no error)"=w428, "waveform name (empty)"="hz" ("group name (empty)"), "group name (empty)"="imaging", "file handle in"=w427) -> ("error out"=w431:errorcluster, "waveform reference"=w432:u32, "file handle out"=w429:u32)  [unwired: 5 in]
              n214 = call-poly <instrlib>:"niHWS Write.vi"("error in (no error)"=w431, "data"=w430, "waveform reference in"=w432) -> ("error out"=w435:errorcluster)  [unwired: 7 in, 1 out]
            }
            frame #1 {
              n215 = call "IMAQ GetImageSize"("Image"=w436, "error in (no error)"=w437) -> ("Y Resolution"=w439:i32, "X Resolution"=w440:i32, "error out"=w438:errorcluster)  [unwired: 2 in]
              n216 = To Double Precision Float(number=w440) -> (double precision float=w441:dbl)
              n217 = Build Array(w441) -> (w442:dbl[])
              n218 = call <instrlib>:"niHWS New Wfm Reference.vi"("error in (no error)"=w438, "waveform name (empty)"="x" ("group name (empty)"), "group name (empty)"="imaging", "file handle in"=w446) -> ("error out"=w444:errorcluster, "waveform reference"=w447:u32, "file handle out"=w445:u32)  [unwired: 5 in]
              n219 = call-poly <instrlib>:"niHWS Write.vi"("error in (no error)"=w444, "data"=w442, "waveform reference in"=w447) -> ("error out"=w443:errorcluster)  [unwired: 7 in, 1 out]
            }
            frame #2 {
              n220 = To Double Precision Float(number=w450) -> (double precision float=w451:dbl)
              n221 = Build Array(w451) -> (w452:dbl[])
              n222 = call <instrlib>:"niHWS New Wfm Reference.vi"("error in (no error)"=w455, "waveform name (empty)"="y" ("group name (empty)"), "group name (empty)"="imaging", "file handle in"=w457) -> ("error out"=w454:errorcluster, "waveform reference"=w460:u32, "file handle out"=w456:u32)  [unwired: 5 in]
              n223 = call-poly <instrlib>:"niHWS Write.vi"("error in (no error)"=w454, "data"=w452, "waveform reference in"=w460) -> ("error out"=w453:errorcluster)  [unwired: 7 in, 1 out]
            }
          }
          n224 = call <instrlib>:"niHWS Close File.vi"("error in (no error)"=w415, "file handle"=w417) -> ("error out"=w426:errorcluster)  [unwired: 9 in]
        }
      }
    }
    frame #3 {
      w552 = T8 3 items=["no dialog", "OK message", "continue or stop message", "OK message + warnings", "continue/stop + warnings"] ("type of dialog (OK msg:1)")
      n225 = invoke on="Recording Path" class="Path" method="Reinit To Default"() -> ()  [unwired: 3 in, 3 out]
      n226 = call <vilib>:"General Error Handler.vi"("type of dialog (OK msg:1)"=w552, "error in (no error)"=w551) -> ()  [unwired: 9 in, 5 out]
    }
  }
